vi "Close file.vi"(8 "error in (no error)":errorcluster, 11 "file refs":T1 {"file" format="%.0x"}) -> (0 "error out":errorcluster)   [LabVIEW 2012]
uses:
  File refs.ctl
  <vilib>/addons/h5labview2/base/hid_t.ctl
  <vilib>/addons/h5labview2/dataset/H5D.lvlib
  <vilib>/addons/h5labview2/file/H5F.lvlib
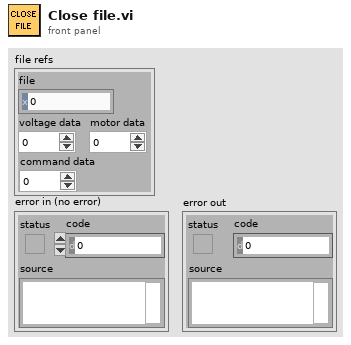
[diagram p1: front panel]
types:
  T1 = typedef "File refs.ctl" = cluster{"file":T2, "voltage data":i32, "motor data":i32, "command data":i32}
  T2 = typedef "hid_t.ctl" = i32
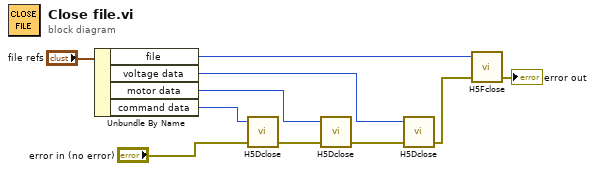
[diagram p0: block diagram]
diagram:
  n1 = Unbundle By Name("file refs") -> ("file"=w9:T2, "voltage data"=w4:i32, "motor data"=w5:i32, "command data"=w6:i32)
  n2 = call <vilib>:"H5Dclose.vi"("error in (no error)"="error in (no error)", "dset in"=w6) -> ("error out"=w2:errorcluster)  [unwired: 3 in]
  n3 = call <vilib>:"H5Dclose.vi"("error in (no error)"=w2, "dset in"=w5) -> ("error out"=w3:errorcluster)  [unwired: 3 in]
  n4 = call <vilib>:"H5Dclose.vi"("error in (no error)"=w3, "dset in"=w4) -> ("error out"=w1:errorcluster)  [unwired: 3 in]
  n5 = call <vilib>:"H5Fclose.vi"("error in (no error)"=w1, "ref"=w9) -> ("error out"=→"error out":errorcluster)  [unwired: 3 in]
